vi "oa_Check Even Angle Output Availability.vi"(8 "error in (no error)":errorcluster, 9 "reached end?":bool, 10 "new signal available?":bool, 11 "segment unit":u16(ring) items=["Time (s)", "Speed (RPM)"]) -> (0 "error out":errorcluster)   [LabVIEW 2017, in "SoundVib_OAUtility.lvlib"]
uses:
  <vilib>/addons/Sound and Vibration/Order Analysis/Utility/SoundVib_OAUtility.lvlib
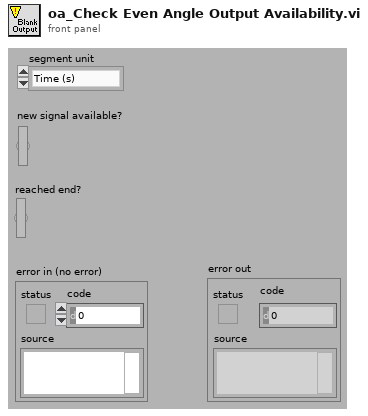
[diagram p1: front panel]
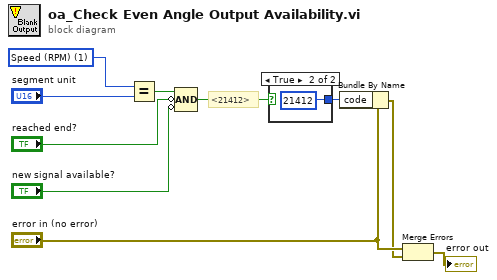
[diagram p0: block diagram]
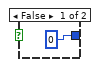
[diagram p2: hidden frame]
diagram:
  w6 = u16 1 items=["Time (s)", "Speed (RPM)"] ("segment unit")
  # "<21412>"
  n1 = Equal?(x=w6, y="segment unit") -> (x = y?=w4:bool)
  n2 = Compound Arithmetic op=AND(w4, invert "reached end?", invert "new signal available?") -> (w1:bool)
  n3 = case shown="True" w1 {
    tunnel: [0 ("code") 21412 ("code")] -> w8
    frame False {
    }
    frame True {
    }
  }
  n4 = Bundle By Name(cluster="error in (no error)", "code"=w8) -> (w7:errorcluster)
  n5 = Merge Errors("error in (no error)", w7) -> (→"error out":errorcluster)
